vi "UpdateComponent.vi"(6 "SymbolIndex(0)":enum16{""}(ring), 8 "error in (no error)":errorcluster, 10 "ComponentName(\"\")":string, 11 "BrowerComponent in":refnum<class "BrowerComponent.lvclass">) -> (0 "error out":errorcluster, 3 "BrowerComponent out":refnum<class "BrowerComponent.lvclass">)   [LabVIEW 2015, in "BrowerComponent.lvclass"]
uses:
  BrowerComponent.lvclass
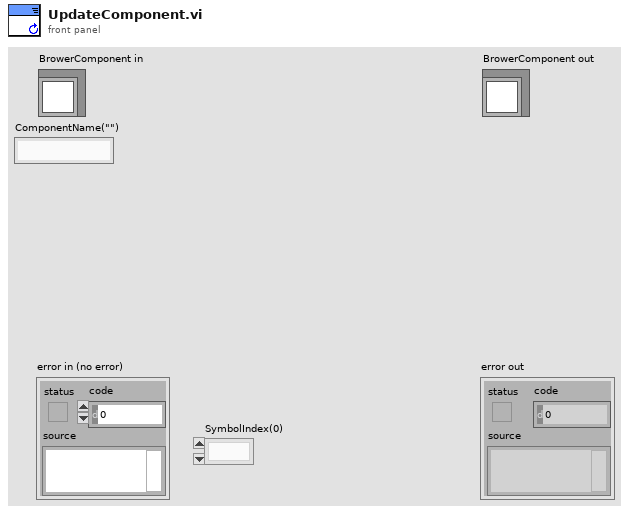
[diagram p1: front panel]
types:
  T1 = typedef "BrowerComponent.lvclass/ObjectAttributes.ctl" = cluster{"ComponentID":string, "SymbolIndex":i32, "ComponentName":string, "PartsOfComponent_dict":variant}
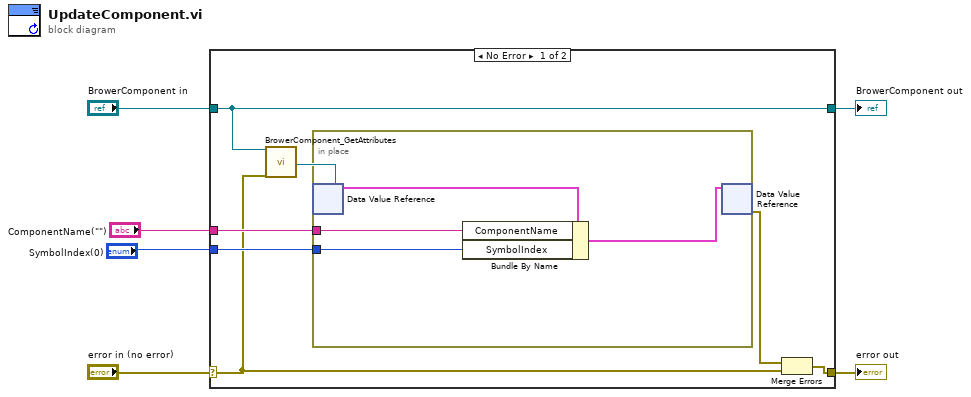
[diagram p0: block diagram]
diagram:
  n1 = case shown="No Error" "error in (no error)" {
    selector: "error in (no error)" -> [w9 w19]
    tunnel: [w7 w19] -> w5
    tunnel: [w13 w18] -> w3
    tunnel: "BrowerComponent in" -> [w13 w18]
    tunnel: "ComponentName(\"\")" -> [w11 _]
    tunnel: "SymbolIndex(0)" -> [w10 _]
    frame No Error {
      n2 = call "BrowerComponent_GetAttributes.vi"("reference in"=w13, "error in (no error)"=w9) -> ("DataRef"=w12:refnum<data-value>)  [unwired: 14 in, 3 out]
      n3 = in-place {
        in-place-border: w11 -> [w16]
        in-place-border: w10 -> [w15]
        n4 = in-place-dvr #1(w12) -> (w17:T1)  [unwired: 1 out]
        n5 = Bundle By Name(cluster=w17, "ComponentName"=w16, "SymbolIndex"=w15) -> (w14:T1)
        n6 = in-place-dvr #1(w14) -> (w8:errorcluster)  [unwired: 1 out]
      }
      n7 = Merge Errors(w8, w9) -> (w7:errorcluster)
    }
    frame Error {
    }
  }
  "error out" <- w5
  "BrowerComponent out" <- w3
